vi "Close Pop-Up (DBL).vi"(8 "error in":errorcluster, 10 "DBL Default":dbl=nan) -> (0 "error out":errorcluster)   [LabVIEW 2021, in "Pop-Up.lvlib" / "Popup.lvclass"]
doc: "This VI can be used to close the pop-up early before the user has finished interacting.\n\nUse this VI to also send a DBL value - this is read when using the Input (DBL) pop-up types.\n\n<b>Code Developed By:</b> +\nDaniel Coons +\nhttps://github.com/danielcoons/tsc-pop-up"
uses:
  Popup.lvclass
  Popup.lvclass/Popup.ctl
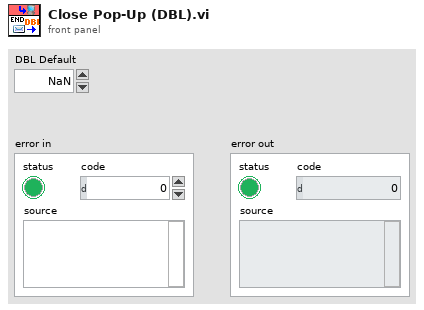
[diagram p1: front panel]
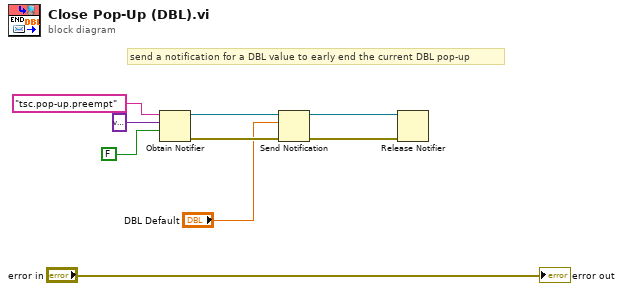
[diagram p0: block diagram]
diagram:
  # "send a notification for a DBL value to early end the current DBL pop-up"
  n1 = Obtain Notifier(name (unnamed)="tsc.pop-up.preempt", notification data type=variant, create if not found? (T)=FALSE) -> (notifier out=w4:refnum<notifier>, error out=w6:errorcluster)  [unwired: 1 in, 1 out]
  n2 = Send Notification(notification="DBL Default", notifier=w4, error in (no error)=w6) -> (notifier out=w3:refnum<notifier>, error out=w5:errorcluster)
  n3 = Release Notifier(notifier=w3, error in (no error)=w5) -> ()  [unwired: 1 in, 3 out]
  "error out" <- "error in"
